vi "Event Messenger Channel Lesson 5.vi"() -> ()   [LabVIEW 2019]
doc: "Lesson 5 combines all the previous lessons in the Event Messenger example and shows a more complex form of messaging feedback from the reader loop to itself."
uses:
  <extravilib>/ChannelInstances/Event Messenger-str/Event Data.ctl
  <extravilib>/ChannelInstances/Event Messenger-u32/Event Data.ctl
  <extravilib>/ChannelInstances/Event Messenger-u32/Instantiate.vi
  <extravilib>/ChannelInstances/Event Messenger-u32/))Channel.vi
  <extravilib>/ChannelInstances/Event Messenger-str/Instantiate.vi
  <extravilib>/ChannelInstances/Event Messenger-str/))Channel.vi
  <extravilib>/ChannelInstances/Event Messenger-str.lvlib
  <extravilib>/ChannelInstances/Event Messenger-u32.lvlib
panel:
  out "Picture":picture
  out "current color":u32(colorbox)
  out "command log":string
  in  "Stop Gamma":bool
  in  "Stop Epsilon":bool
  in  "Stop Beta":bool
  in  "Stop Alpha":bool
  # "Overview: This VI demonstrates how to use the Event Messenger channel wire.\n\nLesson 5 combines all the previous lessons in the Event Messenger example and shows a more complex form of messaging feedback from the reader loop to itself.\n\n\nInstructions:\n1. Run the VI. There are three producers and two consumers, all running at various speeds. Alpha and beta loops produce text commands. Gamma loop produces a color. Delta loop has the job to log all the text commands. Epsilon loop actually does the work of the commands and handles color changes. Epsilon also sends commands to itself, which are properly logged by Delta.\n\n2. Stop the VI by pressing any of the STOP buttons. There will be a slight delay until loop Gamma stops because of its 2 second Wait. \n\n3. Open the block diagram. Review the comments there to see how this VI works."
  # "Producers"
  # "Consumers"
  # "Consumer Delta"
  # "Consumer Epsilon"
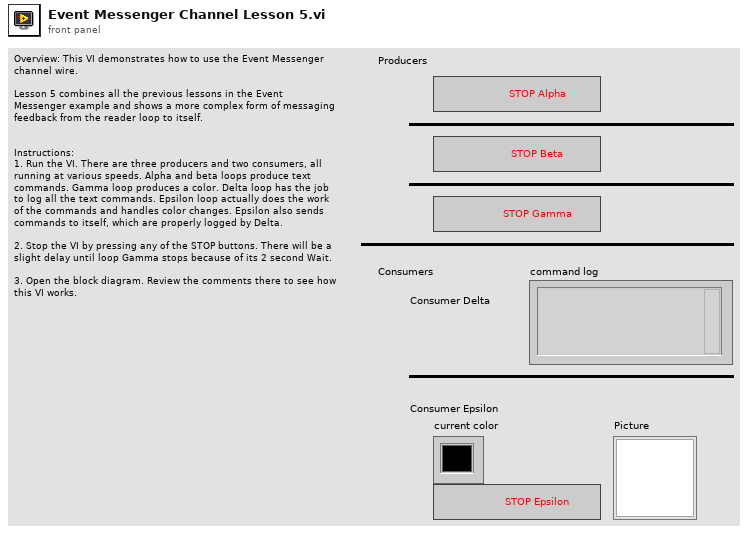
[diagram p1: front panel]
types:
  T1 = cluster{"command":refnum<event-registration>, "new color":refnum<event-registration>}
  T2 = typedef "Event Messenger-str.lvlib/))Channel.ctl" = refnum<queue>
  T3 = typedef "Event Messenger-u32.lvlib/))Channel.ctl" = refnum<queue>
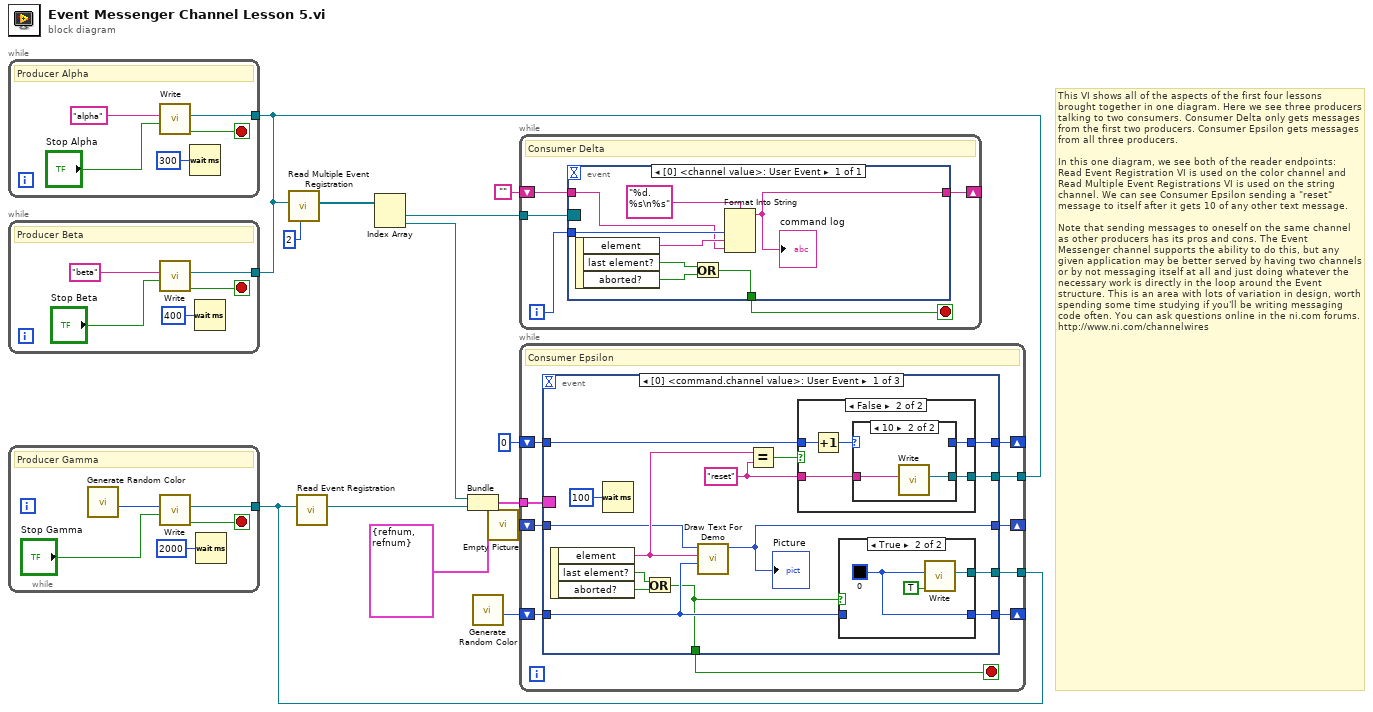
[diagram p0: block diagram]
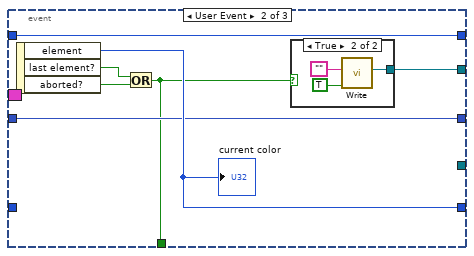
[diagram p5: hidden frame]
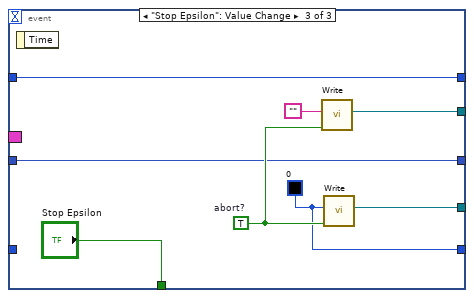
[diagram p7: hidden frame]
diagram:
  # "This VI shows all of the aspects of the first four lessons brought together in one diagram. Here we see three producers talking to two consumers. Consumer Delta only gets messages from the first two producers. Consumer Epsilon gets messages from all three producers.\n\nIn this one diagram, we see both of the reader endpoints: Read Event Registration VI is used on the color channel and Read Multiple Event Registrations VI is used on the string channel. We can see Consumer Epsilon sending a \"reset\" message to itself after it gets 10 of any other text message.\n\nNote that sending messages to oneself on the same channel as other producers has its pros and cons. The Event Messenger channel supports the ability to do this, but any given application may be better served by having two channels or by not messaging itself at all and just doing whatever the necessary work is directly in the loop around the Event structure. This is an area with lots of variation in design, worth spending some time studying if you'll be writing messaging code often. You can ask questions online in the ni.com forums. \nhttp://www.ni.com/channelwires"
  n1 = while {
    tunnel: [w15] -> w12
    stop <- w17 stop-if-true
    # "Producer Beta"
    n2 = call <extravilib>:"Write.vi"("last element? (F)"="Stop Beta", "element"="beta") -> ("done?"=w17:bool, "channel"=w15:T2)  [unwired: 8 in]
    n3 = Wait (ms)(milliseconds to wait=u32 400) -> ()  [unwired: 1 out]
  }
  n4 = while {
    tunnel: w12 -> [w23]
    stop <- w21 stop-if-true
    # "Producer Alpha"
    n5 = call <extravilib>:"Write.vi"("last element? (F)"="Stop Alpha", "element"="alpha") -> ("done?"=w21:bool, "channel"=w23:T2)  [unwired: 8 in]
    n6 = Wait (ms)(milliseconds to wait=u32 300) -> ()  [unwired: 1 out]
  }
  n7 = while {
    tunnel: [w26] -> w6
    stop <- w27 stop-if-true
    # "Producer Gamma"
    n8 = call "Generate Random Color.vi"() -> ("Color"=w24:u32)  [unwired: 11 in]
    n9 = call <extravilib>:"Write.vi"("last element? (F)"="Stop Gamma", "element"=w24) -> ("done?"=w27:bool, "channel"=w26:T3)  [unwired: 8 in]
    n10 = Wait (ms)(milliseconds to wait=u32 2000) -> ()  [unwired: 1 out]
  }
  n11 = call <extravilib>:"Read Multiple Event Registration.vi"("number of event structures"=u16 2 ("# Event structures"), "channel"=w12) -> ("event registration refnums"=w9:refnum<event-registration>[])  [unwired: 9 in]
  n12 = call <extravilib>:"Read Event Registration.vi"("channel"=w6) -> ("event registration refnum"=w7:refnum<event-registration>)  [unwired: 10 in]
  n13 = Index Array(array=w9) -> (element #1=w11:refnum<event-registration>, element #2=w10:refnum<event-registration>)  [unwired: 2 in]
  n14 = Bundle(cluster=T1 {"command"=refnum, "new color"=refnum}, "command"=w10, "new color"=w7) -> (w13:T1)
  n15 = call "Generate Random Color.vi"() -> ("Color"=w5:u32)  [unwired: 11 in]
  n16 = call "Empty Picture"() -> ("empty picture"=w1:picture)
  n17 = while {
    tunnel: w11 -> [w33]
    shift-right: [w29] -> _
    shift-left: "" -> [w31]
    i -> [w30]
    stop <- w32 stop-if-true
    # "Consumer Delta"
    n18 = event shown="[0] <channel value>: User Event" {
      selector: w33 -> [_]
      dyn-events: _ -> [_]
      timeout: _ -> [_]
      tunnel: [w34] -> w32
      tunnel: w31 -> [w38]
      tunnel: w30 -> [w40]
      tunnel: [w37] -> w29
      event User Event {
        n19 = event-data() -> ("element"=w39:string, "last element?"=w36:bool, "aborted?"=w35:bool)  [unwired: 1 in]
        n20 = Or(x=w36, y=w35) -> (x .or. y?=w34:bool)
        n21 = Format Into String(format string="%d. %s\n%s", w40, w39, w38) -> (resulting string=w37:string)  [unwired: 2 in, 1 out]
        "command log" <- w37
      }
    }
  }
  n22 = while {
    tunnel: w13 -> [w50]
    tunnel: w12 -> [w49]
    tunnel: w6 -> [w48]
    shift-right: [w47] -> _
    shift-left: w5 -> [w46]
    shift-right: [w44] -> _
    shift-left: u8 0 -> [w45]
    shift-right: [w43] -> _
    shift-left: w1 -> [w42]
    stop <- w51 stop-if-true
    # "Consumer Epsilon"
    n23 = event shown="[0] <command.channel value>: User Event" {
      selector: w50 -> [_ _ _]
      dyn-events: _ -> [_ _ _]
      timeout: _ -> [_ _ _]
      tunnel: [w52 w80 "Stop Epsilon"] -> w51
      tunnel: [w66 w86 w96] -> w49
      tunnel: [w65 _ w94] -> w48
      tunnel: [w63 w85 w92] -> w47
      tunnel: w46 -> [w58 _ _]
      tunnel: w45 -> [w60 w84 w91]
      tunnel: [w59 w84 w91] -> w44
      tunnel: [w56 w83 w90] -> w43
      tunnel: w42 -> [w55 w83 w90]
      event User Event {
        w61 = "reset" ("element")
        n24 = event-data() -> ("element"=w57:string, "last element?"=w54:bool, "aborted?"=w53:bool)  [unwired: 1 in]
        n25 = Wait (ms)(milliseconds to wait=u32 100) -> ()  [unwired: 1 out]
        n26 = Or(x=w54, y=w53) -> (x .or. y?=w52:bool)
        n27 = call "Draw Text For Demo.vi"("color"=w58, "text"=w57, "picture in"=w55) -> ("picture out"=w56:picture)  [unwired: 8 in]
        "Picture" <- w56
        n28 = Equal?(x=w57, y=w61) -> (x = y?=w62:bool)
        n29 = case shown="False" w62 {
          tunnel: [_ w76] -> w66
          tunnel: w61 -> [_ w75]
          tunnel: w60 -> [w71 w74]
          tunnel: [w71 w72] -> w59
          frame True {
          }
          frame False {
            n30 = Increment(x=w74) -> (x+1=w73:u8)
            n31 = case shown="10" w73 {
              selector: w73 -> [w77 _]
              tunnel: [_ w79] -> w76
              tunnel: w75 -> [_ w78]
              tunnel: [w77 _] -> w72
              frame Default {
              }
              frame 10 {
                n32 = call <extravilib>:"Write.vi"("element"=w78) -> ("channel"=w79:T2)  [unwired: 9 in, 1 out]
              }
            }
          }
        }
        n33 = case shown="True" w52 {
          tunnel: [_ w70] -> w65
          tunnel: [w67 w68] -> w63
          tunnel: w58 -> [w67 _]
          frame False {
          }
          frame True {
            w68 = u32 0 ("random color")
            n34 = call <extravilib>:"Write.vi"("abort (F)"=TRUE ("element valid? (T)"), "element"=w68) -> ("channel"=w70:T3)  [unwired: 8 in, 1 out]
          }
        }
      }
      event User Event {
        n35 = event-data() -> ("element"=w85:u32, "last element?"=w81:bool, "aborted?"=w82:bool)  [unwired: 1 in]
        "current color" <- w85
        n36 = Or(x=w81, y=w82) -> (x .or. y?=w80:bool)
        n37 = case shown="True" w80 {
          tunnel: [_ w89] -> w86
          frame False {
          }
          frame True {
            n38 = call <extravilib>:"Write.vi"("abort (F)"=TRUE ("element valid? (T)"), "element"="") -> ("channel"=w89:T2)  [unwired: 8 in, 1 out]
          }
        }
      }
      event "Stop Epsilon": Value Change {
        w92 = u32 0 ("random color")
        w95 = TRUE  # abort?
        n39 = event-data() -> ()  [unwired: 1 in, 1 out]
        n40 = call <extravilib>:"Write.vi"("abort (F)"=w95, "element"="") -> ("channel"=w96:T2)  [unwired: 8 in, 1 out]
        n41 = call <extravilib>:"Write.vi"("abort (F)"=w95, "element"=w92) -> ("channel"=w94:T3)  [unwired: 8 in, 1 out]
      }
    }
  }
